vi "Solenoid_PanelSim_Global.vi"(0 "Menu":T3=enum."delete", 5 "Channel":i32, 7 "Boolean Value":bool, 9 "Numeric Value":dbl format="%#.4f", 11 "error in (no error)":errorcluster, 12 "String Value":string) -> (10 "Value out":T1={"type"="Solenoid", "device"="", "name"="", "data"={"<output"=FALSE}}, 15 "error out":errorcluster)   [LabVIEW 2019]
doc: "This is used to set and get the last motor output values. This is needed for simulation, since we cannot read these values from the hardware.\n\nThis software is licensed. Open the labview\\readme\\WPI Robotics Library Open Source License.txt file for more information."
uses:
  Solenoid Data proto.ctl
  Solenoid proto.ctl
  Solenoid Update Ops.ctl
panel:
  out "All Values":T1[](array[typedef])
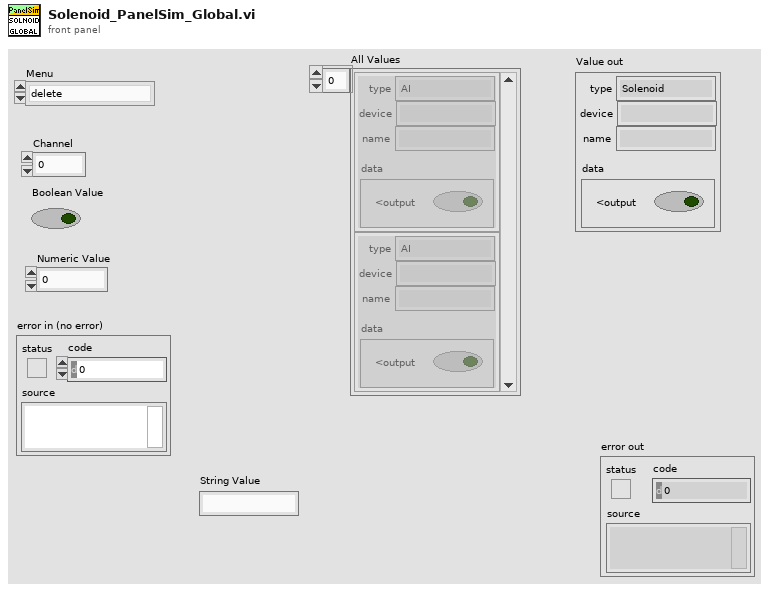
[diagram p1: front panel]
types:
  T1 = typedef "Solenoid proto.ctl" = cluster{"type":string, "device":string, "name":string, "data":T2}
  T2 = typedef "Solenoid Data proto.ctl" = cluster{"<output":bool}
  T3 = typedef "Solenoid Update Ops.ctl" = enum16{"get", "delete", "JSON update", "set  name", "transmit initial", "reset", "set init", "set output"}
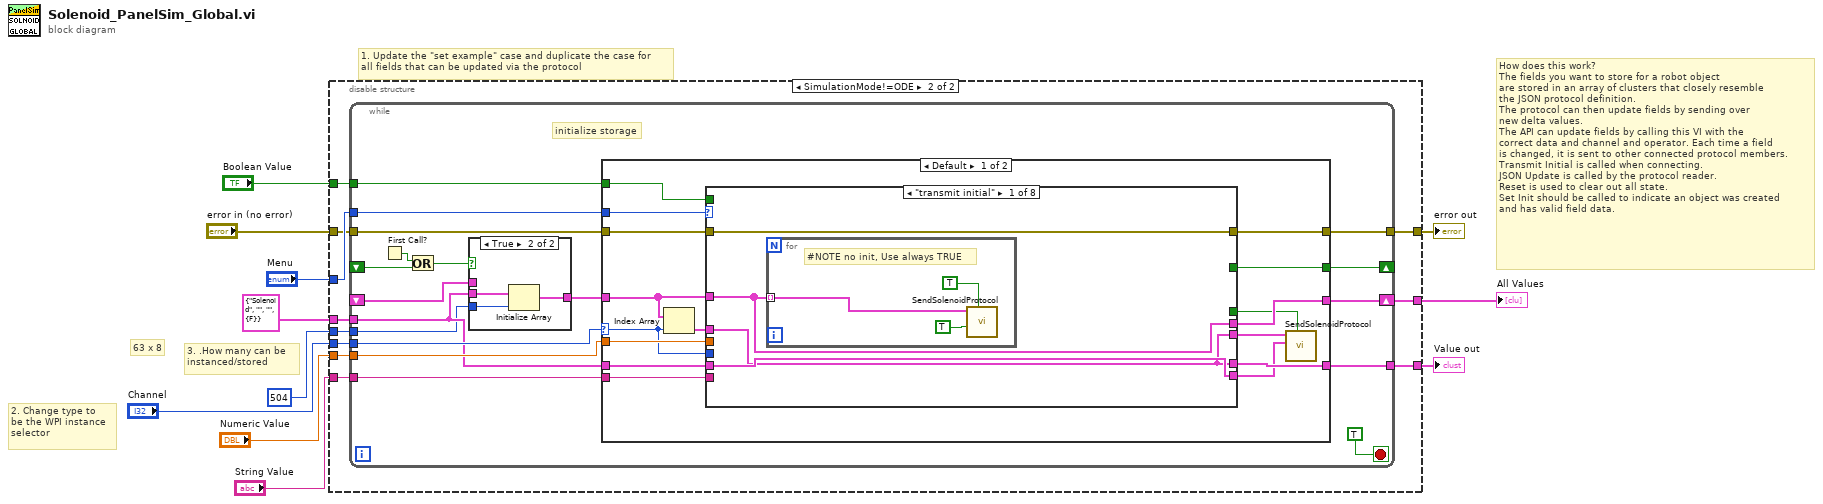
[diagram p0: block diagram]
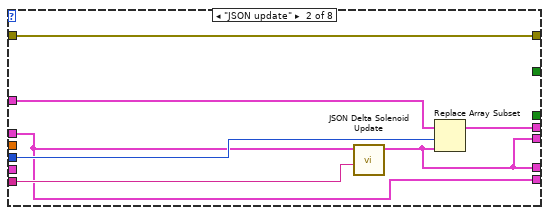
[diagram p3: hidden frame]
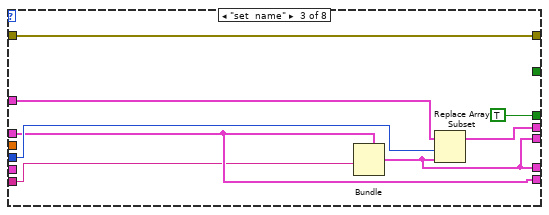
[diagram p4: hidden frame]
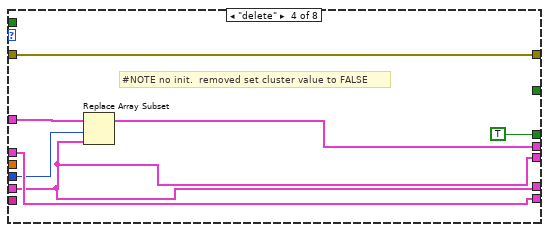
[diagram p5: hidden frame]
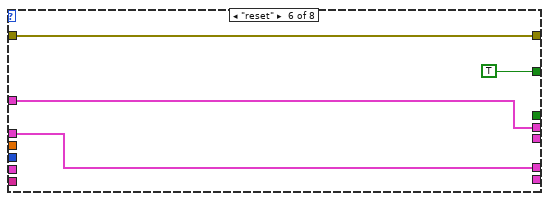
[diagram p7: hidden frame]
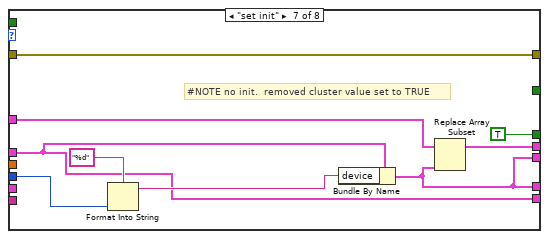
[diagram p8: hidden frame]
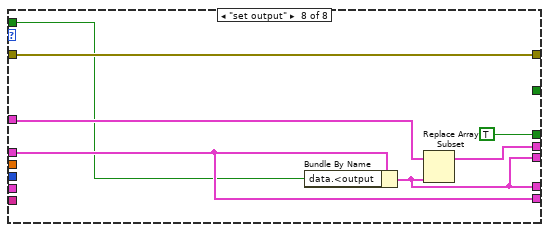
[diagram p9: hidden frame]
diagram:
  # "63 x 8"
  # "How does this work?\nThe fields you want to store for a robot object\nare stored in an array of clusters that closely resemble\nthe JSON protocol definition.\nThe protocol can then update fields by sending over\nnew delta values.\nThe API can update fields by calling this VI with the\ncorrect data and channel and operator. Each time a field\nis changed, it is sent to other connected protocol members.\nTransmit Initial is called when connecting.\nJSON Update is called by the protocol reader.\nReset is used to clear out all state.\nSet Init should be called to indicate an object was created\nand has valid field data."
  # "1. Update the \"set example\" case and duplicate the case for\nall fields that can be updated via the protocol"
  # "2. Change type to\nbe the WPI instance\nselector"
  # "3. .How many can be\ninstanced/stored"
  n1 = disable-structure shown="SimulationMode!=ODE" {
    disable-tunnel: "Menu" -> [_ w24]
    disable-tunnel: [w13 w23] -> w10
    disable-tunnel: "error in (no error)" -> [w13 w22]
    disable-tunnel: [_ w21] -> w8
    disable-tunnel: "Numeric Value" -> [_ w20]
    disable-tunnel: "Channel" -> [_ w19]
    disable-tunnel: [w12 w18] -> w5
    disable-tunnel: T1 {"type"="Solenoid", "device"="", "name"="", "data"={"<output"=FALSE}} ("Accel value out") -> [w12 w17]
    disable-tunnel: "String Value" -> [_ w16]
    disable-tunnel: 504 -> [_ w15]
    disable-tunnel: "Boolean Value" -> [_ w14]
    frame condition #0 {
    }
    frame condition #1 (active) {
      n2 = while {
        tunnel: w20 -> [w42]
        tunnel: w22 -> [w38]
        shift-right: [w41] -> w21
        shift-left: _ -> [w34]
        tunnel: [w40] -> w18
        tunnel: w24 -> [w39]
        tunnel: [w37] -> w23
        tunnel: w19 -> [w33]
        tunnel: w17 -> [w32]
        tunnel: w16 -> [w31]
        shift-right: [w27] -> _
        shift-left: _ -> [w28]
        tunnel: w15 -> [w26]
        tunnel: w14 -> [w25]
        stop <- TRUE stop-if-true
        # "initialize storage"
        n3 = First Call?() -> (First Call?: T/F=w29:bool)
        n4 = Or(x=w29, y=w28) -> (x .or. y?=w30:bool)
        n5 = case shown="True" w30 {
          tunnel: [w114 w117] -> w35
          tunnel: w34 -> [w114 _]
          tunnel: w32 -> [_ w116]
          tunnel: w26 -> [_ w115]
          frame False {
          }
          frame True {
            n6 = Initialize Array(w116, w115) -> (w117:T1[])
          }
        }
        n7 = case shown="Default" w33 {
          selector: w33 -> [w51 _]
          tunnel: w42 -> [w58 _]
          tunnel: [w57 w113] -> w41
          tunnel: [w56 w111] -> w40
          tunnel: w39 -> [w55 _]
          tunnel: w38 -> [w54 w112]
          tunnel: [w53 w112] -> w37
          tunnel: w35 -> [w52 w113]
          tunnel: w32 -> [w49 w111]
          tunnel: w31 -> [w48 _]
          tunnel: [w47 _] -> w27
          tunnel: w25 -> [w43 _]
          frame Default {
            n8 = Index Array(array=w52, index=w51) -> (element=w50:T1)
            n9 = case shown="\"transmit initial\"" w55 {
              tunnel: w58 -> [_ _ _ _ _ _ _ _]
              tunnel: [w59 w72 w80 w86 w90 w94 w99 w108] -> w57
              tunnel: w52 -> [w59 w70 w78 w87 w90 w94 w98 w109]
              tunnel: [w60 w68 w73 w81 w88 w92 w96 w105] -> w56
              tunnel: [w62 w71 w79 w85 w89 w93 w95 w110] -> w53
              tunnel: w54 -> [w62 w71 w79 w85 w89 w93 w95 w110]
              tunnel: w51 -> [_ w69 w76 w82 _ _ w102 _]
              tunnel: [w60 w68 w73 w81 _ _ w96 w105] -> w45
              tunnel: [w61 w66 w75 w83 _ _ w97 w106] -> w44
              tunnel: [_ _ TRUE TRUE _ _ TRUE TRUE] -> w46
              tunnel: w50 -> [w60 w66 w75 w83 w88 w92 w97 w106]
              tunnel: w49 -> [w61 _ _ w81 _ _ _ _]
              tunnel: w48 -> [_ w67 w74 _ _ _ _ _]
              tunnel: [_ _ _ _ _ TRUE _ _] -> w47
              tunnel: w43 -> [_ _ _ _ _ _ _ w104]
              frame "transmit initial" {
                n10 = for {
                  tunnel: w59 -> [w65] mode=indexing
                  # "#NOTE no init, Use always TRUE"
                  n11 = call "SendSolenoidProtocol.vi"("Send"=TRUE, "Initialize"=TRUE ("Send"), "Current"=w65) -> ()  [unwired: 9 in]
                }
              }
              frame "JSON update" {
                n12 = call "JSON Delta Solenoid Update.vi"("Delta JSON"=w67, "input"=w66) -> ("output"=w68:T1)  [unwired: 8 in, 1 out]
                n13 = Replace Array Subset(array=w70, new element=w68, index=w69) -> (w72:T1[])
              }
              frame "set  name" {
                n14 = Bundle(cluster=w75, "name"=w74) -> (w73:T1)  [unwired: 3 in]
                n15 = Replace Array Subset(array=w78, new element=w73, index=w76) -> (w80:T1[])
              }
              frame "delete" {
                # "#NOTE no init.  removed set cluster value to FALSE"
                n16 = Replace Array Subset(array=w87, new element=w81, index=w82) -> (w86:T1[])
              }
              frame "get" {
              }
              frame "reset" {
              }
              frame "set init" {
                # "#NOTE no init.  removed cluster value set to TRUE"
                n17 = Format Into String(format string="%d", w102) -> (resulting string=w101:string)  [unwired: 2 in, 1 out]
                n18 = Bundle By Name(cluster=w97, "device"=w101) -> (w96:T1)
                n19 = Replace Array Subset(array=w98, new element=w96) -> (w99:T1[])  [unwired: 1 in]
              }
              frame "set output" {
                n20 = Bundle By Name(cluster=w106, "data.<output"=w104) -> (w105:T1)
                n21 = Replace Array Subset(array=w109, new element=w105) -> (w108:T1[])  [unwired: 1 in]
              }
            }
            n22 = call "SendSolenoidProtocol.vi"("Send"=w46, "Previous"=w44, "Current"=w45) -> ()  [unwired: 9 in]
          }
          frame -1 {
            # "Do nothing if \nchannel is Invalid."
          }
        }
      }
    }
  }
  "error out" <- w10
  "Value out" <- w5
  "All Values" <- w8
